vi "Check Test Identification.vi"(8 "error in (no error)":errorcluster, 11 "Test Identification":T1) -> (0 "error out":errorcluster, 3 "Continue?":bool)   [LabVIEW 2016]
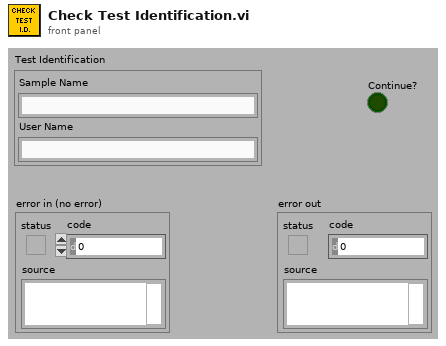
[diagram p1: front panel]
types:
  T1 = cluster{"Sample Name":string, "User Name":string}
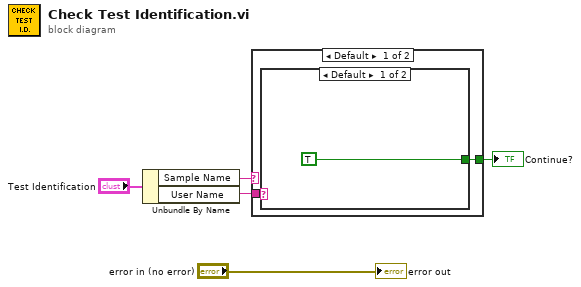
[diagram p0: block diagram]
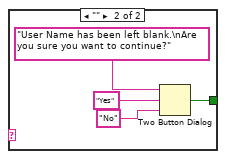
[diagram p2: hidden frame]
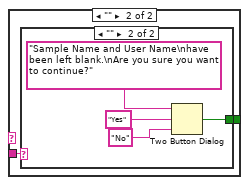
[diagram p3: hidden frame]
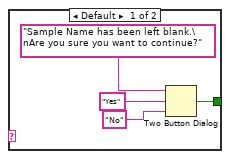
[diagram p4: hidden frame]
diagram:
  n1 = Unbundle By Name("Test Identification") -> ("Sample Name"=w4:string, "User Name"=w5:string)
  n2 = case shown="Default" w4 {
    tunnel: w5 -> [w7 w14]
    tunnel: [w6 w13] -> w1
    frame Default {
      n3 = case shown="Default" w7 {
        tunnel: [TRUE ("T button?") w9] -> w6
        frame Default {
        }
        frame "" {
          n4 = Two Button Dialog(message="User Name has been left blank.\nAre you sure you want to continue?", 1:"No" ("F button name (\"Cancel\")"), 2:"Yes" ("T button name (\"OK\")")) -> (T button?=w9:bool)
        }
      }
    }
    frame "" {
      n5 = case shown="\"\"" w14 {
        tunnel: [w15 w19] -> w13
        frame Default {
          n6 = Two Button Dialog(message="Sample Name has been left blank.\nAre you sure you want to continue?", 1:"No" ("F button name (\"Cancel\")"), 2:"Yes" ("T button name (\"OK\")")) -> (T button?=w15:bool)
        }
        frame "" {
          n7 = Two Button Dialog(message="Sample Name and User Name\nhave been left blank.\nAre you sure you want to continue?", 1:"No" ("F button name (\"Cancel\")"), 2:"Yes" ("T button name (\"OK\")")) -> (T button?=w19:bool)
        }
      }
    }
  }
  "Continue?" <- w1
  "error out" <- "error in (no error)"
